vi "Main_Stagefright.vi"() -> ()   [LabVIEW 2012]
uses:
  <vilib>/vision/Image Controls.llb/IMAQ Image.ctl
  <vilib>/vision/NI_Vision_Development_Module.lvlib
panel:
  out "FileVersion":string
  out "Position.y":sgl format="%#.0f"
  out "Position.x":sgl format="%#.0f"
  out "Score":sgl format="%#.0f"
  out "Fiducial Template":T1(plugin-control)
  out "Score all":sgl[](array[numeric])=[207.96088, 1000.0, 164.13931, 159.61043, 129.57571, 190.89413, 153.79263, 159.79875, 217.61157, 150.5897, 141.03848, 539.2585, 523.24445, 511.9799, 522.9404, 526.40063, 548.3722, 524.07715, 509.34766, 529.9397, 530.2488, 546.94275, 528.6569, 540.79004, 501.09125, 521.29175]
  in  "Fiducial Template":string(combo)="Template_20x_sobel.png"
  in  "Save results to CSV":bool
  out "Filename":variant=variant(refnum<image> "StageFrightChip_20x2.bmp")
  out "Source Images":T1[](array[plugin-control])=["20x.bmp", "20x_sobel.bmp", "StageFrightChip_20x.bmp", "StageFrightChip_20x1.bmp", "StageFrightChip_20x2.bmp", "StageFrightChip_20x3.bmp", "StageFrightChip_20x4.bmp", "StageFrightChip_20x5.bmp", "StageFrightChip_20x6.bmp", "StageFrightChip_20x7.bmp", "StageFrightChip_20x8.bmp", "StageFrightChip_20x_sobel.bmp", "StageFrightChip_20x_sobel1.bmp", "StageFrightChip_20x_sobel2.bmp", "StageFrightChip_20x_sobel3.bmp", "StageFrightChip_20x_sobel4.bmp", "StageFrightChip_20x_sobel5.bmp", "StageFrightChip_20x_sobel6.bmp", "StageFrightChip_20x_sobel7.bmp", "StageFrightChip_20x_sobel8.bmp", "StageFrightChip_20x_sobelBright1.bmp", "StageFrightChip_20x_sobelBright2.bmp", "StageFrightChip_20x_sobelBright3.bmp", "StageFrightChip_20x_sobelBright4.bmp", "StageFrightChip_20x_sobelBright5.bmp", "StageFrightChip_20x_sobelBright6.bmp"]
  in  "Size":sgl=10.0
  out "PosY":sgl[](array[numeric])=[1066.1215, 935.5, 484.42477, 541.02295, 617.27484, 638.56024, 1321.046, 729.54535, 897.5891, 1030.7277, 1241.2319, 849.8333, 683.0109, 688.1466, 792.6854, 966.86365, 1146.5382, 1156.1758, 744.771, 868.2035, 868.9183, 866.75134, 866.2604, 1187.9204, 417.75464, 416.24948]
  out "PosX":sgl[](array[numeric])=[1098.6714, 1030.0, 1410.8555, 1155.8539, 1625.7227, 334.02856, 229.2192, 1038.1204, 937.4752, 1740.9315, 435.25806, 1455.6796, 1458.8976, 810.25146, 1064.1396, 1065.0979, 1443.9667, 421.36115, 418.361, 1327.8506, 1331.1934, 1539.8466, 316.55002, 318.59637, 315.33258, 1460.1486]
  in  "Find Patterns":bool
  in  "Folder for Analysis (BMP)":path=path "C:/Users/kevinsh/Desktop/Fiducial Training"
  in  "Overlay Color":u32(colorbox)=16711680
  out "All Results":T1(plugin-control)
  in  "Rotation Angle \nSearch Ranges":cluster{"Start":sgl, "End":sgl}[](array[cluster])=[{"Start"=-10.0, "End"=10.0}]
  in  "Minimum Match Score":sgl=100.0
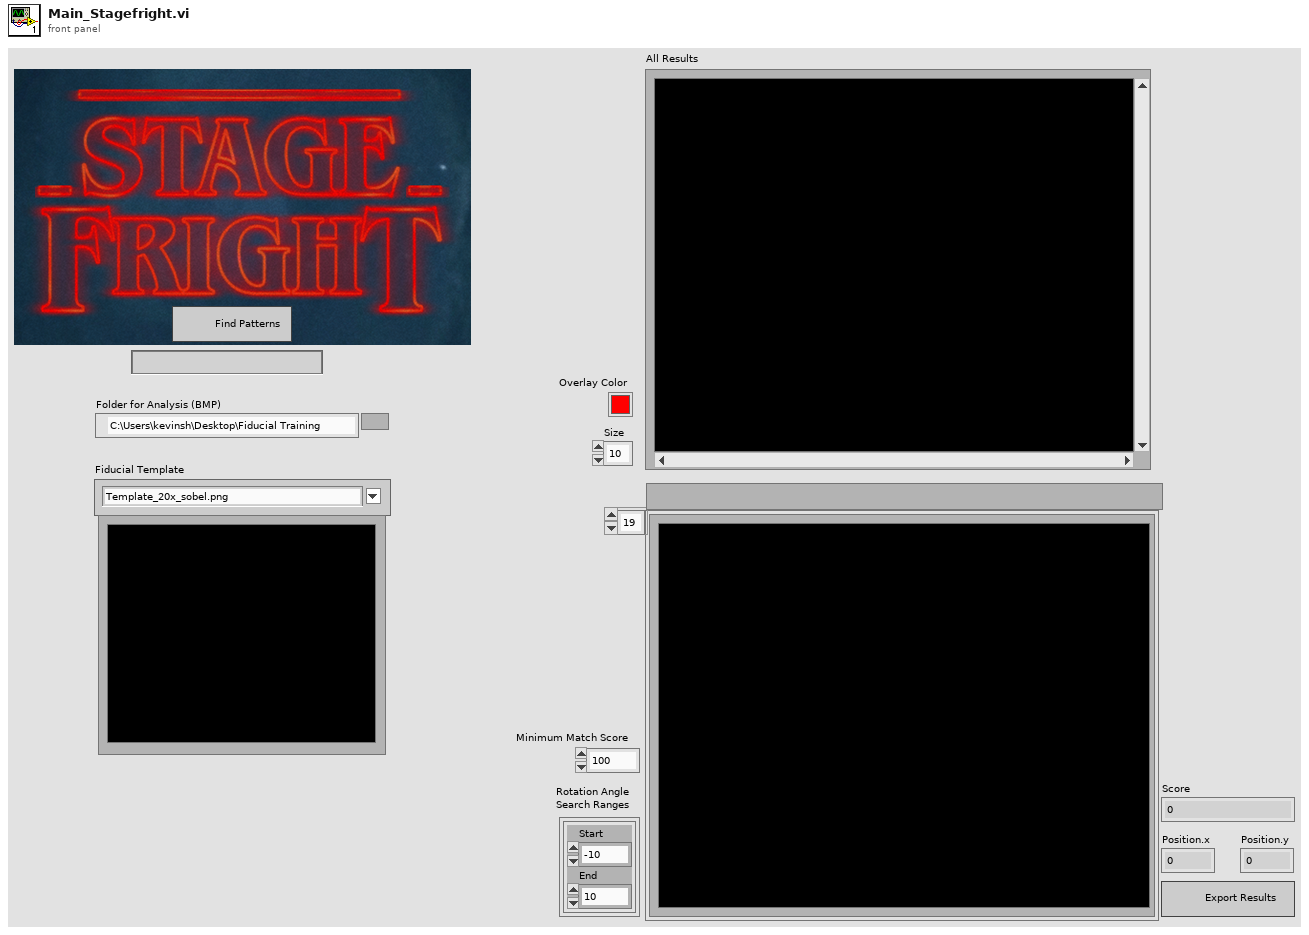
[diagram p1: front panel]
types:
  T1 = typedef "IMAQ Image.ctl" = refnum<image>
  T2 = enum32{"invalid app kind", "Development System", "Run Time System", "Student Edition", "Embedded LabVIEW", "Evaluation", "Custom"}
  T3 = enum32{"Invalid", "Standard", "Closed", "Hidden", "Minimized", "Maximized"}
  T4 = cluster{"Match Mode":u16, "Number of Matches Requested":i32, "Minimum Match Score":sgl, "SubPixel Accuracy":bool, "Rotation Angle Ranges":cluster{"Start":sgl, "End":sgl}[], "Show Search Area":bool, "Show Result":bool}
  T5 = cluster{"Core":cluster{"Current VI Reference":refnum<vi>, "Close Panel on Exit?":bool}, "FiducialImages":T1[], "ImageResults":T1, "PatternTemplate":T1, "PosX":sgl[], "PosY":sgl[], "Score":sgl[], "Folder for Analysis":path, "filenames for processing":string[], "Fiducial Template Path":path, "Data Export Filepath":path}
  T6 = typedef "Image Type" = u32
  T7 = cluster{"Current VI Reference":refnum<vi>, "Close Panel on Exit?":bool}
  T8 = cluster{"Position":cluster{"x":sgl, "y":sgl}, "Angle":sgl, "Scale":sgl, "Score":sgl, "Bounding Box":cluster{"x":sgl, "y":sgl}[]}[]
  T9 = cluster{"Position":cluster{"x":sgl, "y":sgl}, "Angle":sgl, "Scale":sgl, "Score":sgl, "Bounding Box":cluster{"x":sgl, "y":sgl}[]}
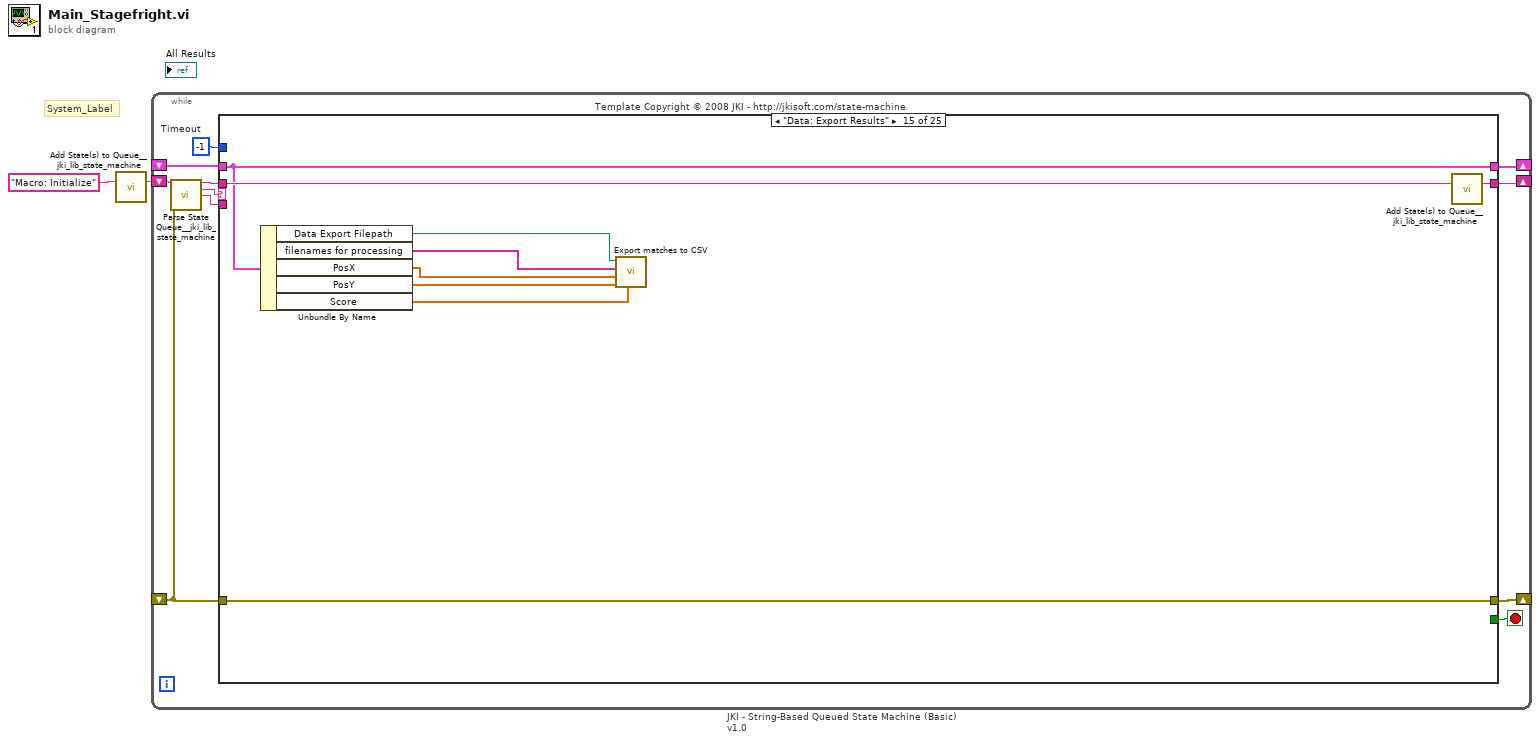
[diagram p0: block diagram]
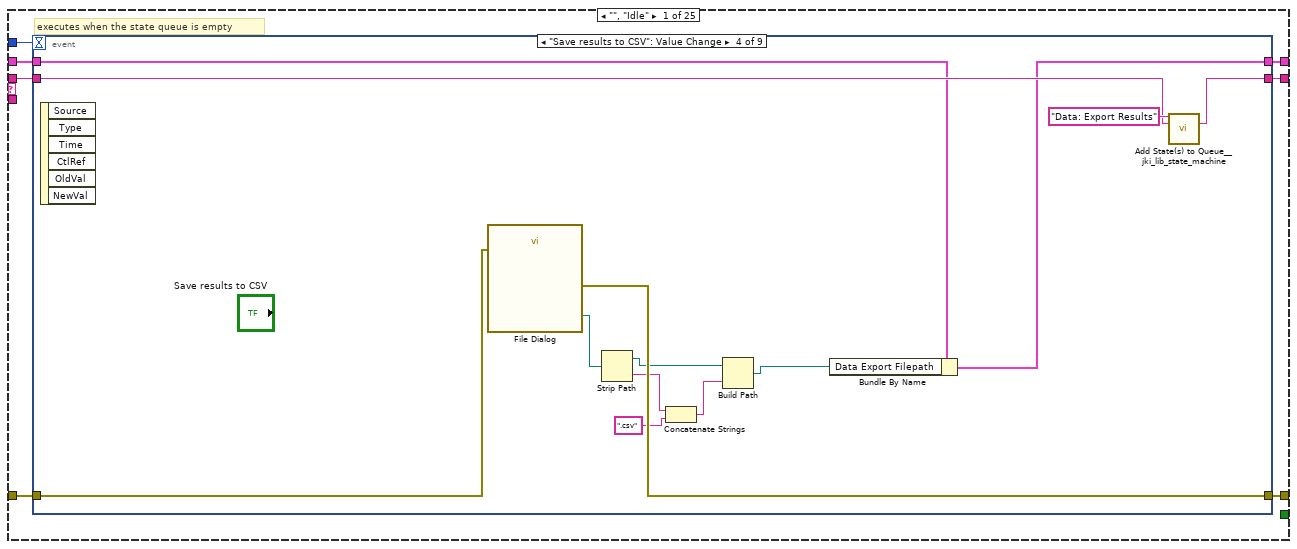
[diagram p2: hidden frame]
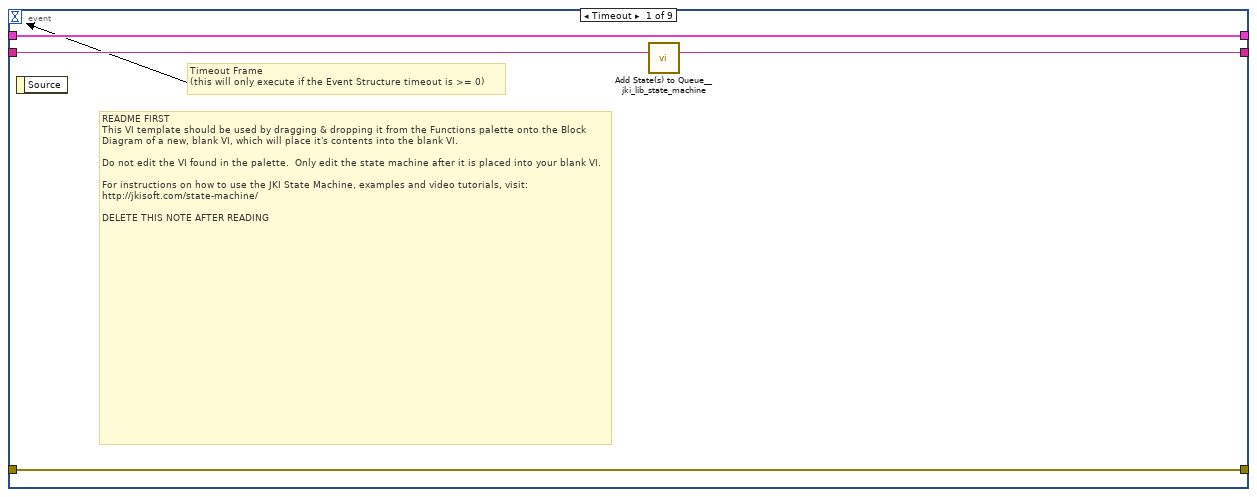
[diagram p3: hidden frame]
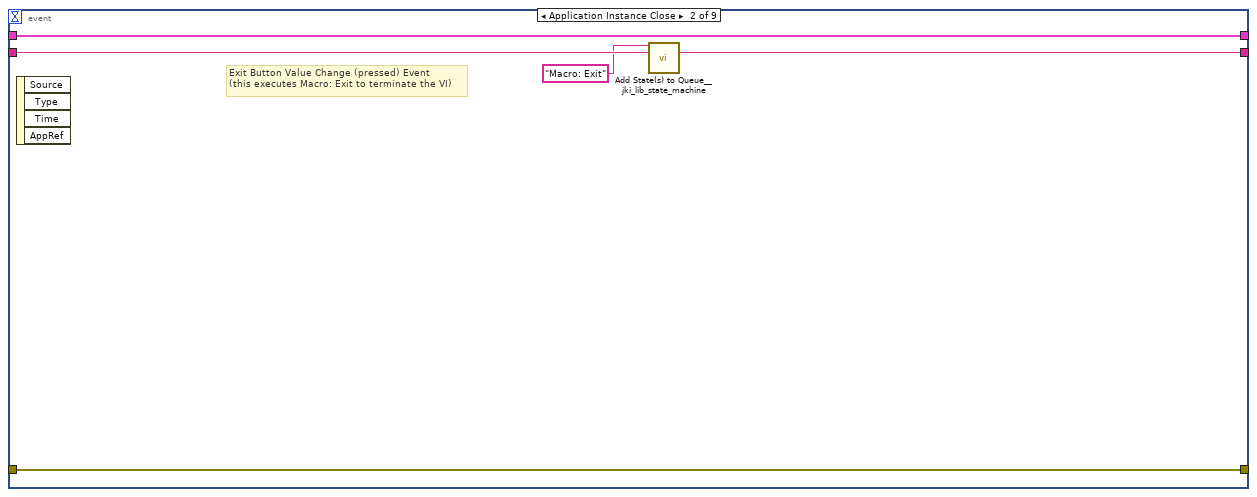
[diagram p4: hidden frame]
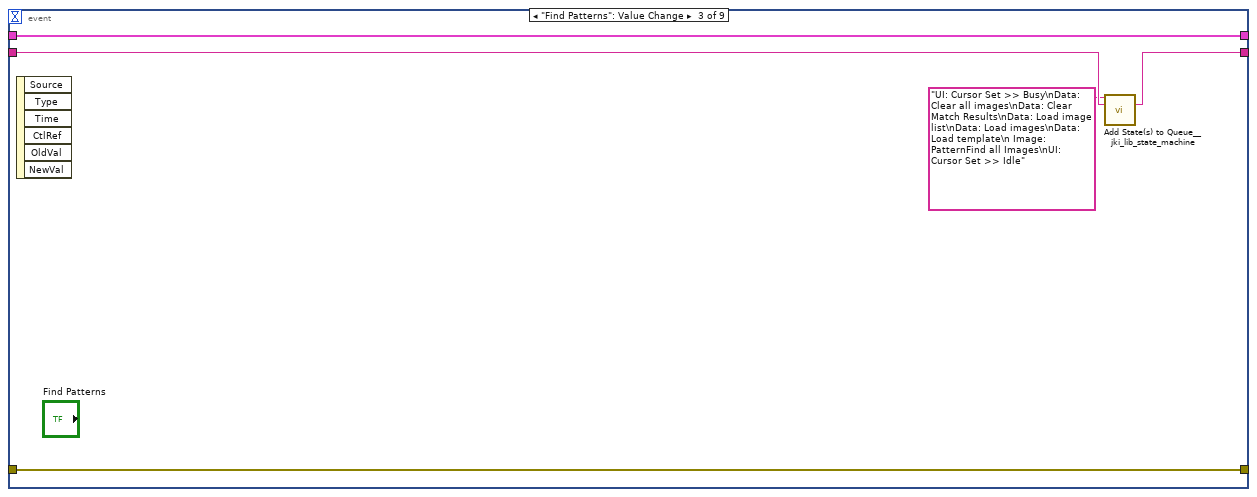
[diagram p5: hidden frame]
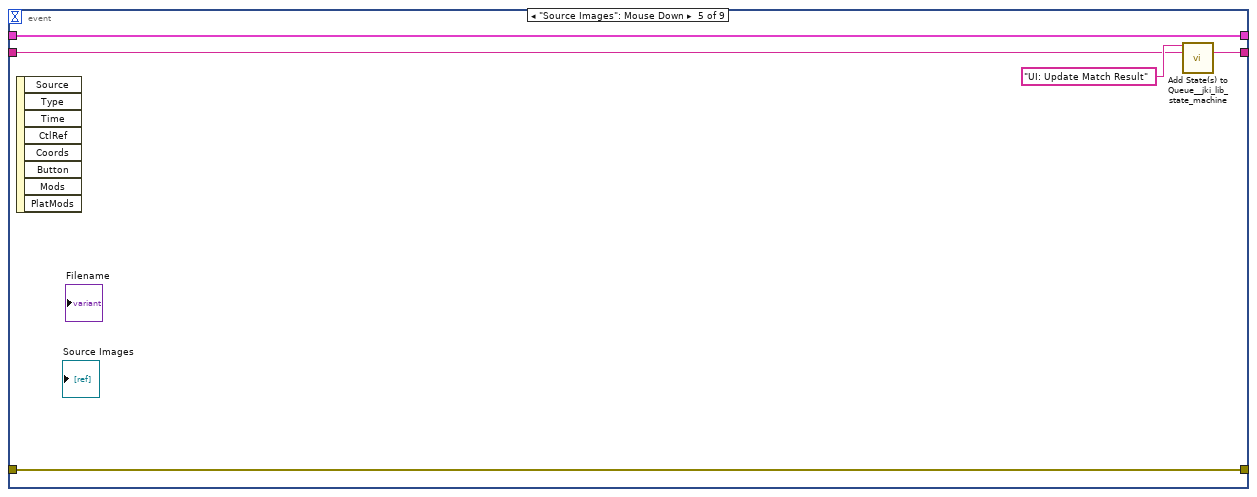
[diagram p6: hidden frame]
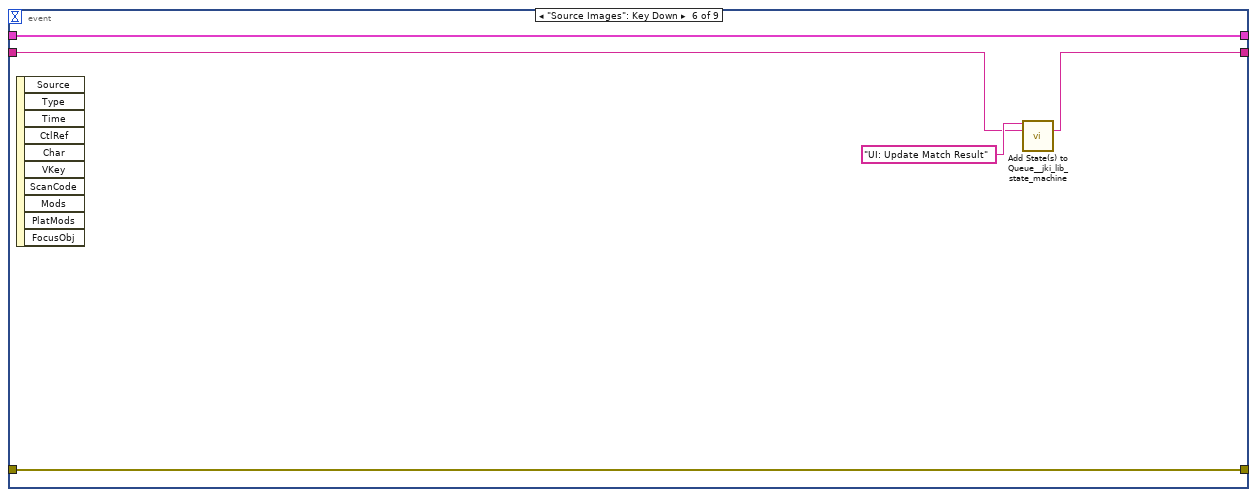
[diagram p7: hidden frame]
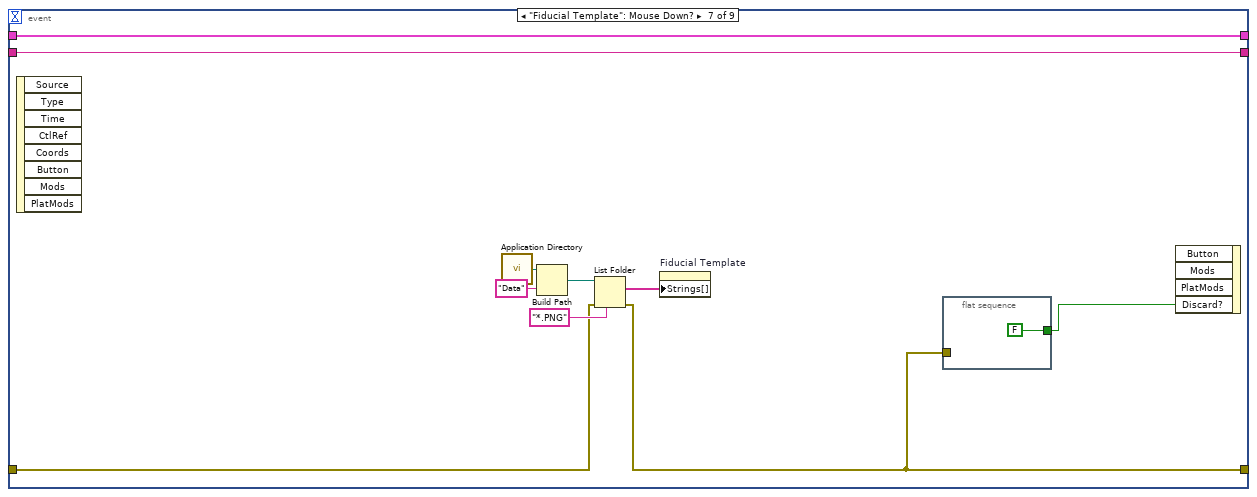
[diagram p8: hidden frame]
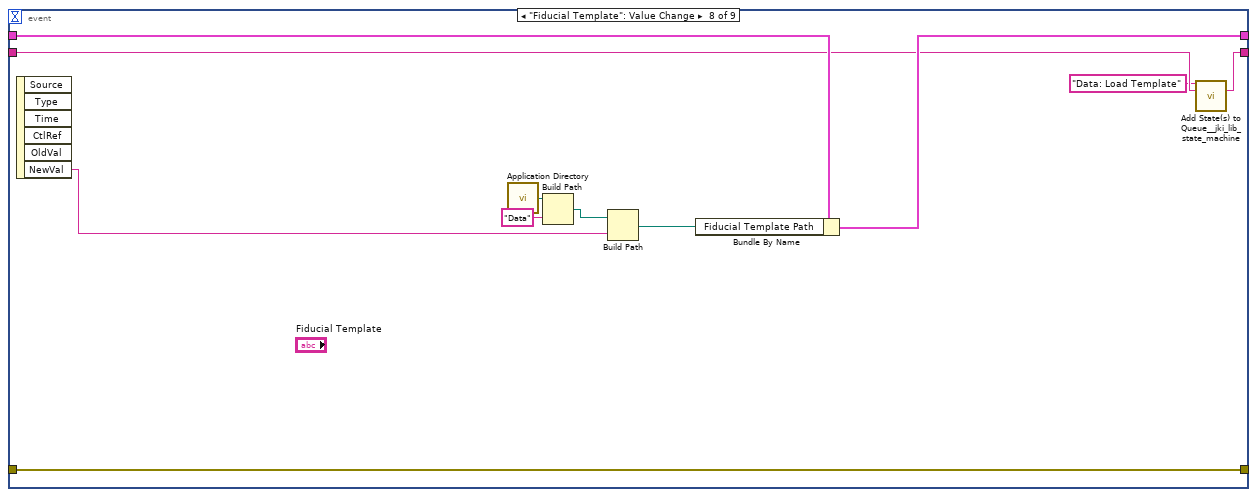
[diagram p9: hidden frame]
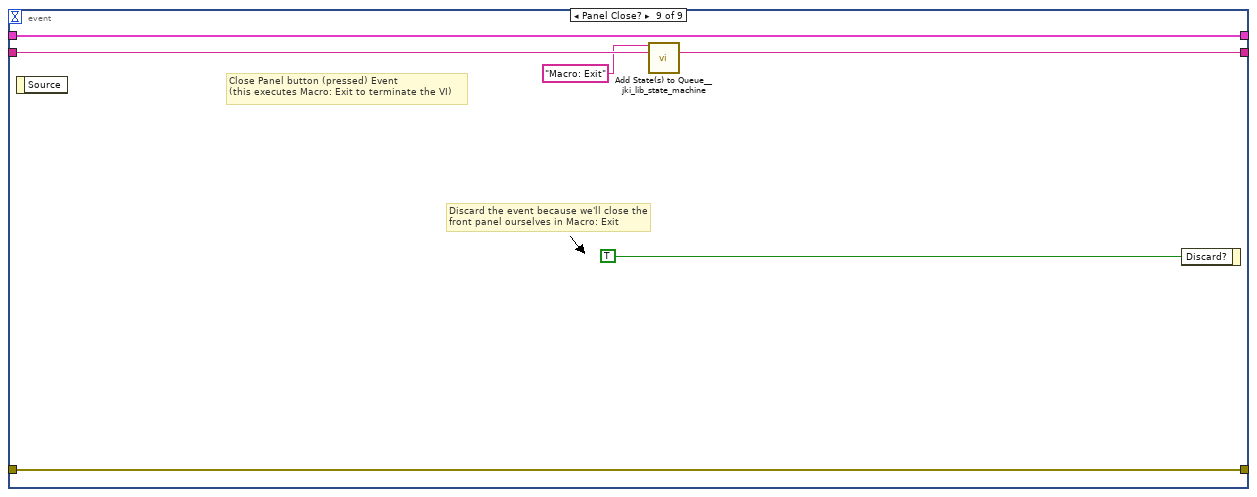
[diagram p10: hidden frame]
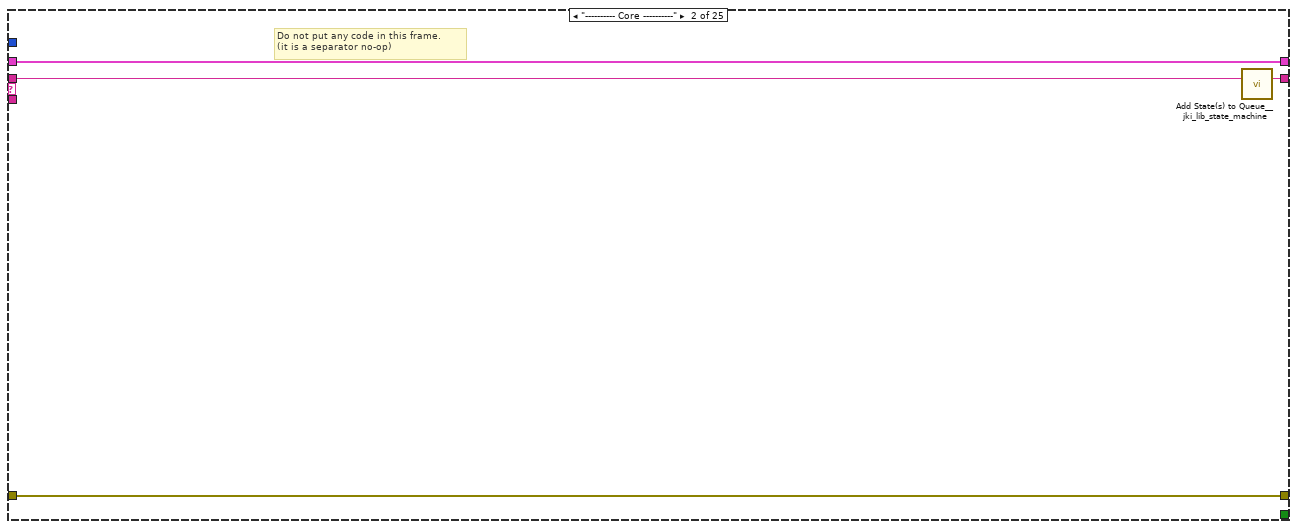
[diagram p11: hidden frame]
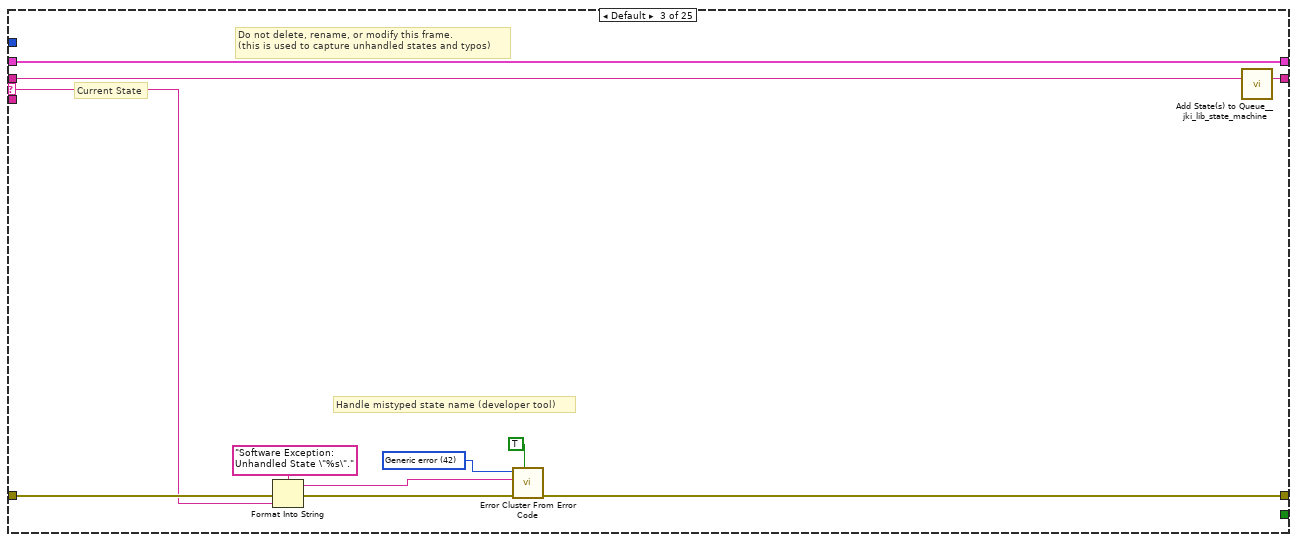
[diagram p12: hidden frame]
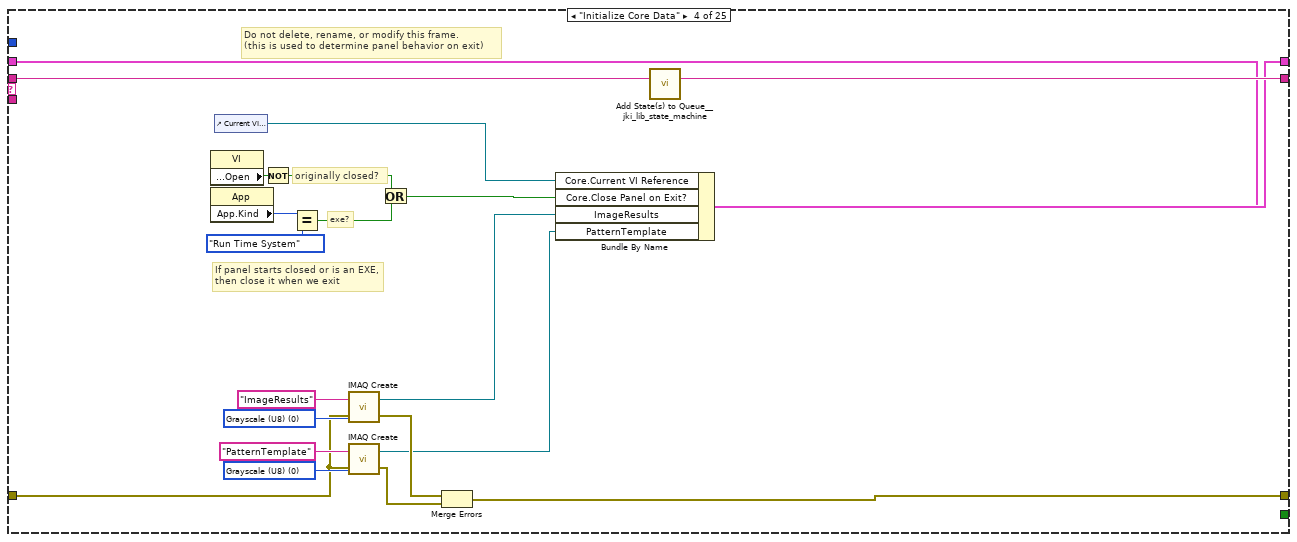
[diagram p13: hidden frame]
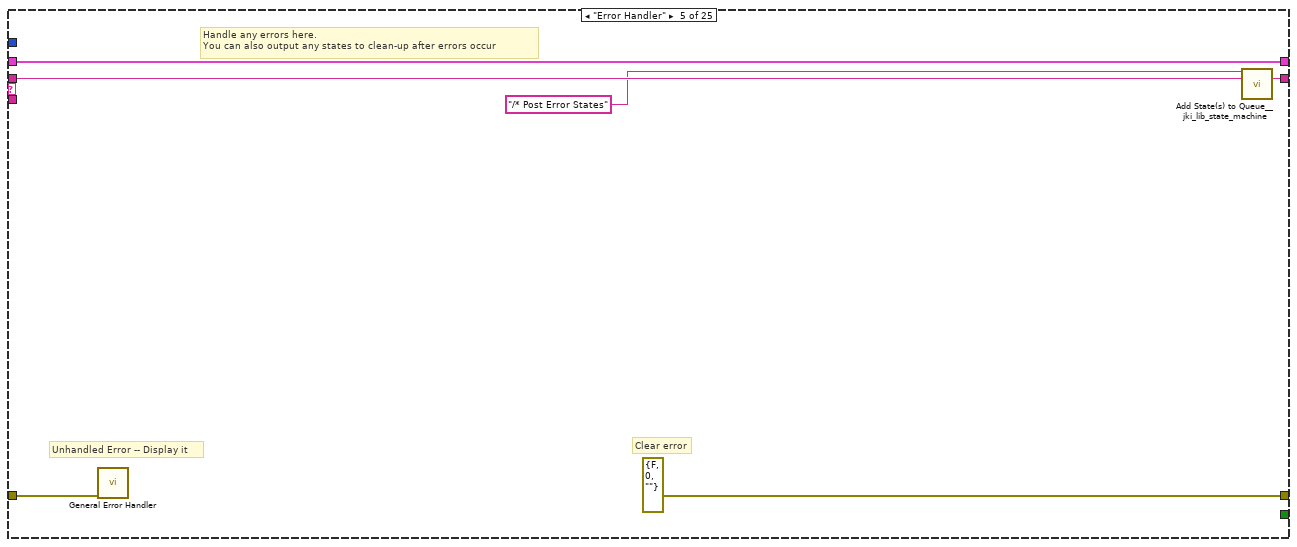
[diagram p14: hidden frame]
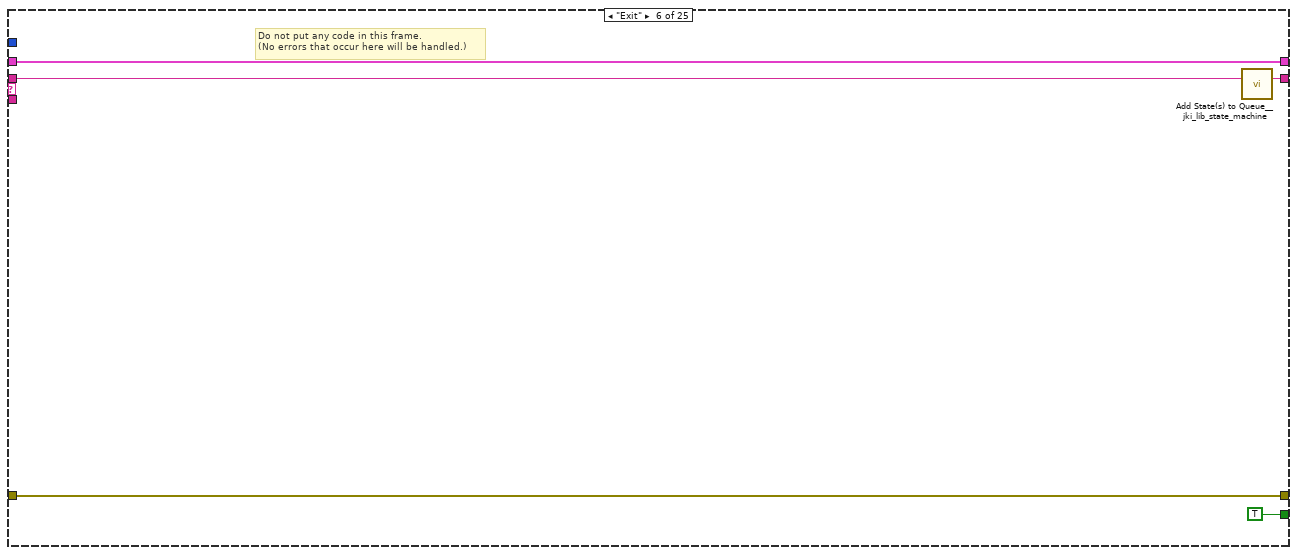
[diagram p15: hidden frame]
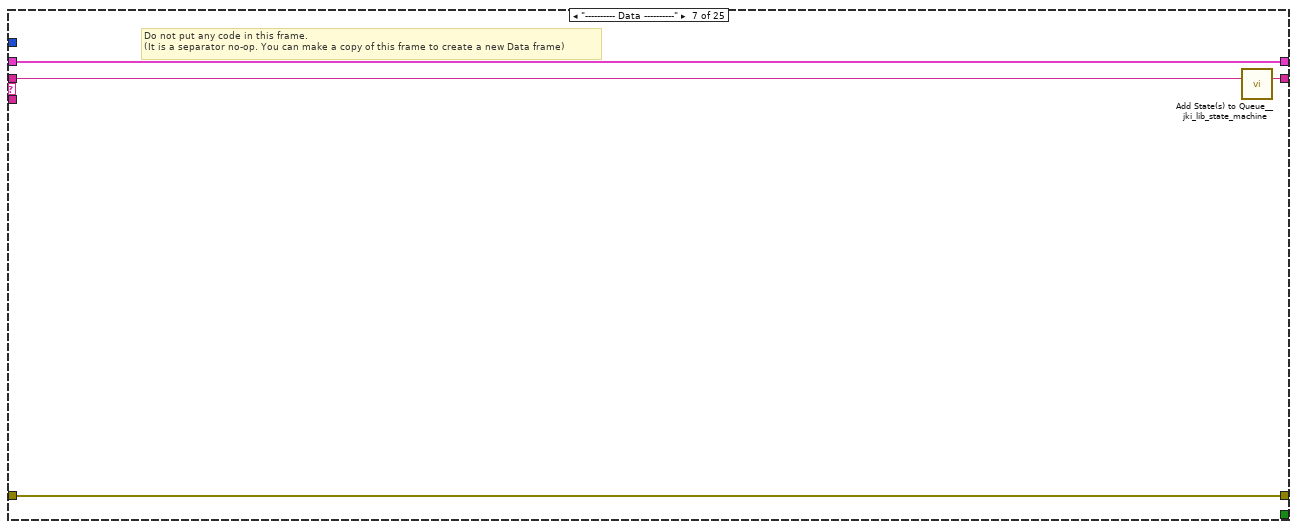
[diagram p16: hidden frame]
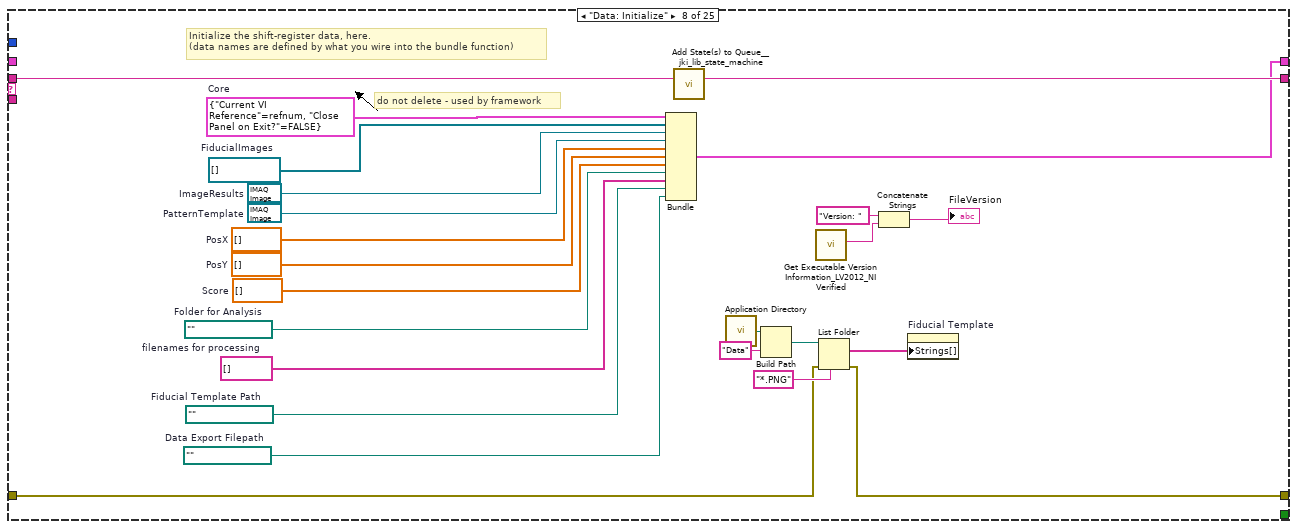
[diagram p17: hidden frame]
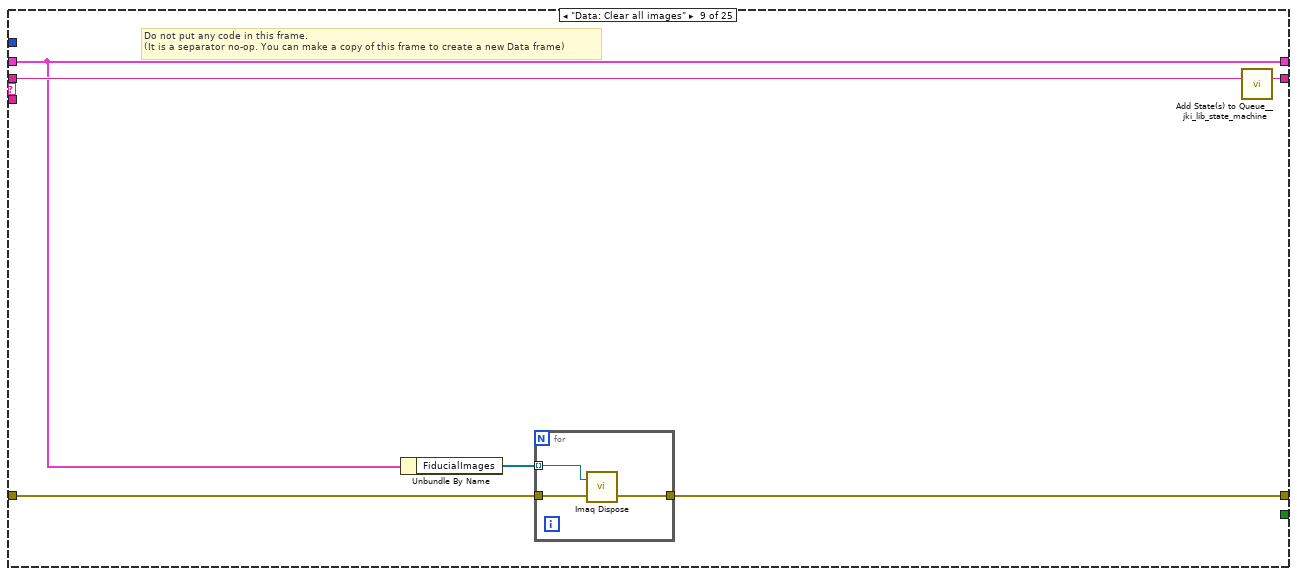
[diagram p18: hidden frame]
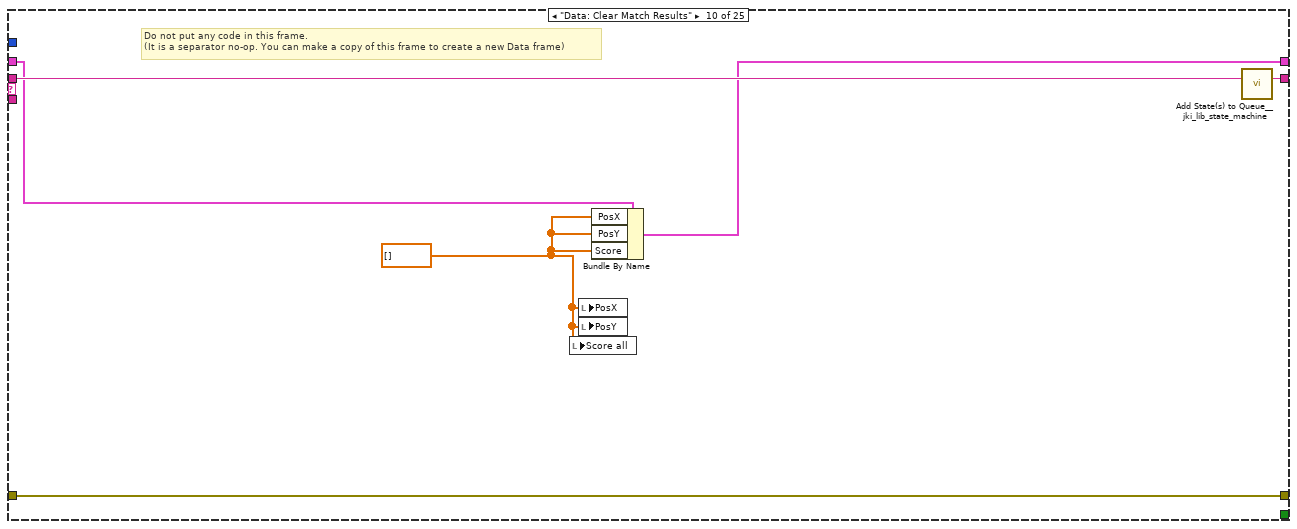
[diagram p19: hidden frame]
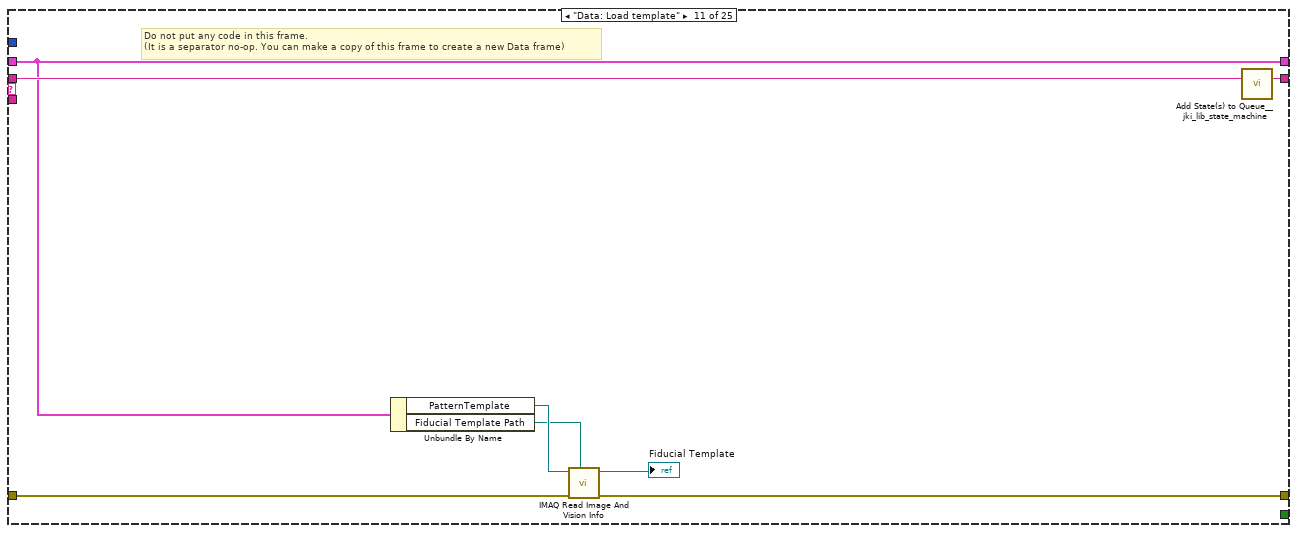
[diagram p20: hidden frame]
diagram:
  # "System_Label"
  n1 = call <vilib>:"Add State(s) to Queue__jki_lib_state_machine.vi"("State(s) in (\"\")"="Macro: Initialize") -> ("States Out"=w2:string)  [unwired: 14 in]
  n2 = while "JKI - String-Based Queued State Machine (Basic) v1.0" {
    shift-right: [w6] -> _
    shift-left: _ -> [w5]
    shift-right: [w9] -> _
    shift-left: _ -> [w3]
    shift-right: [w8] -> _
    shift-left: w2 -> [w10]
    stop <- w7 stop-if-true
    w4 = -1  # Timeout
    # "Template Copyright © 2008 JKI - http://jkisoft.com/state-machine"
    n3 = call <vilib>:"Parse State Queue__jki_lib_state_machine.vi"("State Queue"=w10, "Error In (no error)"=w3) -> ("Remaining States"=w12:string, "Current State"=w13:string, "Arguments"=w11:string)  [unwired: 11 in]
    n4 = case shown="\"Data: Export Results\"" w13 {
      selector: w13 -> [_ _ w90 _ _ _ _ _ _ _ _ _ _ _ _ _ _ _ _ _ _ _ _ _ _]
      tunnel: w12 -> [w20 w89 w94 w121 w127 w132 w136 w160 w166 w175 w183 w192 w204 w222 w231 w235 w248 w252 w258 w269 w295 w300 w310 w314 w335]
      tunnel: w11 -> [_ _ _ _ _ _ _ _ _ _ _ _ _ _ _ _ _ _ w253 w263 _ _ _ _ _]
      tunnel: w5 -> [w18 w86 w92 w113 w124 w130 w133 _ w162 w172 w180 w185 w199 w218 w228 w232 w243 w250 w256 w265 w292 w297 w307 w311 w331]
      tunnel: [w17 w87 w96 w102 errorcluster {"status"=FALSE, "code"=0, "source"=""} ("error out") w129 w134 w143 w163 w173 w178 w186 w196 w219 w229 w233 w246 w249 w254 w266 w293 w298 w308 w312 w325] -> w9
      tunnel: w3 -> [w16 w87 w95 w105 w123 w129 w134 w144 w164 w173 w179 w187 w202 w216 w229 w233 w246 w249 w255 w267 w293 w298 w308 w312 w333]
      tunnel: [w19 w88 w93 w120 w126 w131 w135 w159 w165 w174 w182 w191 w203 w221 w230 w234 w247 w251 w257 w268 w294 w299 w309 w313 w334] -> w8
      tunnel: [_ _ _ _ _ TRUE _ _ _ _ _ _ _ _ _ _ _ _ _ _ _ _ _ _ _] -> w7
      tunnel: [w15 w86 w92 w119 w124 w130 w133 w158 w162 w171 w180 w184 w198 w218 w228 w232 w243 w250 w256 w265 w292 w297 w307 w311 w329] -> w6
      tunnel: w4 -> [w14 _ _ _ _ _ _ _ _ _ _ _ _ _ _ _ _ _ _ _ _ _ _ _ _]
      frame "", "Idle" {
        # "executes when the state queue is empty"
        n5 = event shown="[3] \"Save results to CSV\": Value Change" {
          selector: _ -> [_ _ _ _ _ _ _ _ _]
          dyn-events: _ -> [_ _ _ _ _ _ _ _ _]
          timeout: w14 -> [_ _ _ _ _ _ _ _ _]
          tunnel: w20 -> [w24 w29 w32 w46 w49 w54 w67 w70 w85]
          tunnel: [w23 w28 w31 w45 w48 w53 w67 w71 w84] -> w19
          tunnel: w18 -> [w21 w26 w33 w42 w51 w56 w66 w77 w82]
          tunnel: [w22 w27 w34 w43 w52 w57 w58 w79 w83] -> w17
          tunnel: w16 -> [w22 w27 w34 w44 w52 w57 w60 w79 w83]
          tunnel: [w21 w26 w33 w41 w51 w56 w66 w76 w82] -> w15
          event Timeout {
            # "README FIRST\nThis VI template should be used by dragging & dropping it from the Functions palette onto the Block Diagram of a new, blank VI, which will place it's contents into the blank VI.\n\nDo not edit the VI found in the palette.  Only edit the state machine after it is placed into your blank VI.\n\nFor instructions on how to use the JKI State Machine, examples and video tutorials, visit:\nhttp://jkisoft.com/state-machine/\n\nDELETE THIS NOTE AFTER READING"
            # "Timeout Frame\n(this will only execute if the Event Structure timeout is >= 0)"
            n6 = event-data() -> ()  [unwired: 1 in, 1 out]
            n7 = call <vilib>:"Add State(s) to Queue__jki_lib_state_machine.vi"("State(s) in (\"\")"=w24) -> ("States Out"=w23:string)  [unwired: 14 in]
          }
          event Application Instance Close {
            # "Exit Button Value Change (pressed) Event\n(this executes Macro: Exit to terminate the VI)"
            n8 = event-data() -> ()  [unwired: 1 in, 4 out]
            n9 = call <vilib>:"Add State(s) to Queue__jki_lib_state_machine.vi"("State(s) in Front (\"\")"="Macro: Exit", "State(s) in (\"\")"=w29) -> ("States Out"=w28:string)  [unwired: 13 in]
          }
          event "Find Patterns": Value Change {
            n10 = event-data() -> ()  [unwired: 1 in, 6 out]
            n11 = call <vilib>:"Add State(s) to Queue__jki_lib_state_machine.vi"("State(s) in Front (\"\")"="UI: Cursor Set >> Busy\nData: Clear all images\nData: Clear Match Results\nData: Load image list\nData: Load images\nData: Load template\n Image: PatternFind all Images\nUI: Cursor Set >> Idle" ("State(s) in Front (\"\")"), "State(s) in (\"\")"=w32) -> ("States Out"=w31:string)  [unwired: 13 in]
          }
          event "Save results to CSV": Value Change {
            n12 = event-data() -> ()  [unwired: 1 in, 6 out]
            n13 = call "File Dialog"("error in"=w44) -> ("selected path"=w40:path, "error out"=w43:errorcluster)  [unwired: 11 in, 2 out]
            n14 = Strip Path(path=w40) -> (stripped path=w39:path, name=w38:string)
            n15 = Concatenate Strings(w38, ".csv" ("name or relative path")) -> (w36:string)
            n16 = Build Path(base path=w39, name or relative path=w36) -> (appended path=w35:path)
            n17 = Bundle By Name(cluster=w42, "Data Export Filepath"=w35) -> (w41:T5)
            n18 = call <vilib>:"Add State(s) to Queue__jki_lib_state_machine.vi"("State(s) in Front (\"\")"="Data: Export Results" ("State(s) in Front (\"\")"), "State(s) in (\"\")"=w46) -> ("States Out"=w45:string)  [unwired: 13 in]
          }
          event "Source Images": Mouse Down {
            n19 = event-data() -> ()  [unwired: 1 in, 8 out]
            n20 = call <vilib>:"Add State(s) to Queue__jki_lib_state_machine.vi"("State(s) in Front (\"\")"="UI: Update Match Result", "State(s) in (\"\")"=w49) -> ("States Out"=w48:string)  [unwired: 13 in]
          }
          event "Source Images": Key Down {
            n21 = event-data() -> ()  [unwired: 1 in, 10 out]
            n22 = call <vilib>:"Add State(s) to Queue__jki_lib_state_machine.vi"("State(s) in Front (\"\")"="UI: Update Match Result", "State(s) in (\"\")"=w54) -> ("States Out"=w53:string)  [unwired: 13 in]
          }
          event "Fiducial Template": Mouse Down? {
            n23 = event-data() -> ()  [unwired: 1 in, 8 out]
            n24 = call <vilib>:"Application Directory.vi"() -> ("Application Directory"=w64:path)
            n25 = Build Path(base path=w64, name or relative path="Data") -> (appended path=w65:path)
            n26 = List Folder(path=w65, pattern="*.PNG", error in=w60) -> (filenames=w62:string[], error out=w58:errorcluster)  [unwired: 1 in, 2 out]
            n27 = property on="Fiducial Template" class="CmbBox"("Strings[]"=w62) -> ()  [unwired: 2 in, 2 out]
            n28 = flat-sequence {
              tunnel: [FALSE ("Discard?")] -> w59
              tunnel: w58 -> [_]
              frame #0 {
              }
            }
            n29 = event-data("Discard?"=w59) -> ()  [unwired: 4 in, 1 out]
          }
          event "Fiducial Template": Value Change {
            n30 = event-data() -> ("NewVal"=w78:string)  [unwired: 1 in, 5 out]
            n31 = call <vilib>:"Application Directory.vi"() -> ("Application Directory"=w74:path)
            n32 = Build Path(base path=w74, name or relative path="Data") -> (appended path=w72:path)
            n33 = Build Path(base path=w72, name or relative path=w78) -> (appended path=w75:path)
            n34 = Bundle By Name(cluster=w77, "Fiducial Template Path"=w75) -> (w76:T5)
            n35 = call <vilib>:"Add State(s) to Queue__jki_lib_state_machine.vi"("State(s) in Front (\"\")"="Data: Load Template" ("State(s) in Front (\"\")"), "State(s) in (\"\")"=w70) -> ("States Out"=w71:string)  [unwired: 13 in]
          }
          event Panel Close? {
            # "Discard the event because we'll close the front panel ourselves in Macro: Exit"
            # "Close Panel button (pressed) Event\n(this executes Macro: Exit to terminate the VI)"
            n36 = event-data() -> ()  [unwired: 1 in, 1 out]
            n37 = call <vilib>:"Add State(s) to Queue__jki_lib_state_machine.vi"("State(s) in Front (\"\")"="Macro: Exit", "State(s) in (\"\")"=w85) -> ("States Out"=w84:string)  [unwired: 13 in]
            n38 = event-data("Discard?"=TRUE) -> ()  [unwired: 1 in, 1 out]
          }
        }
      }
      frame "---------- Core ----------" {
        # "Do not put any code in this frame.\n(it is a separator no-op)"
        n39 = call <vilib>:"Add State(s) to Queue__jki_lib_state_machine.vi"("State(s) in (\"\")"=w89) -> ("States Out"=w88:string)  [unwired: 14 in]
      }
      frame Default {
        w99 = 42 items=["No error", "Argument error", "Memory is full", "Out of zone", "End of file", "File already open", "Generic file I/O error", "File not found", "File permission error", "Disk is full", "Duplicate path", "Too many files open", "System feature not enabled", "Resource file not found", "Cannot add resource", "Resource not found", "Image not found", "Image memory error", "Pen does not exist", "Config type invalid", "Config token not found", "Config parse error", "Config memory error", "Bad external code format", "Bad external code offset", "External code not present", "Null window", "Destroy window error", "Null menu", "Print aborted", "Bad print record", "Print driver error", "Windows error during printing", "Memory error during printing", "Print dialog error", "Generic print error", "Invalid device refnum", "Device not found", "Device parameter error", "Device unit error", "Cannot open device", "Device call aborted", "Generic error", "Cancelled by user", "Object ID too low", "Object ID too high", "Object not in heap", "Unknown heap", "Unknown object (invalid DefProc)", "Unknown object (DefProc not in table)", "Message out of range", "Invalid (null) method", "Unknown message", "Manager call not supported", "Bad address", "Network operation in progress", "Network operation timed out", "Connection is busy", "Network attribute not supported", "Network error", "Address in use", "System out of memory", "Connection aborted", "Connection refused", "Not connected", "Already connected", "Connection closed", "Initialization error (interapplication manager)", "Bad occurrence", "Wait on unbound occurrence handler", "Occurrence queue overflow", "Datalog type conflict", "Unused", "Unrecognized type (interapplication manager)", "Memory corrupt", "Failed to make temporary DLL", "Old CIN version", "Drag socket not found", "Failed to load drop-object", "Failed to register OLE object", "Failed to release OLE object", "Format specifier type mismatch", "Unknown format specifier", "Too few format specifiers", "Too many format specifiers", "Scan failed", "Newer CIN version", "Error converting to variant", "Runtime menu error", "Password tampered", "Variant attribute not found", "Incompatible variant data type", "Event data is not available", "Event Store is not present", "Occurrence is not found", "Event Queue is not created", "Event info is not available", "Refnum passed is NULL", "Error retrieving Class GUID", "Error retrieving CoClass GUID", "Error retrieving TypeLib GUID.", "Bad built application magic bytes.", "Specific driver is different from the specific driver associated with the Logical Name.", "There is no session opened to the class driver.", "Max Error", "MAX - Error with config objects", "MAX - Error loading configuration", "MAX - Group not supported"]
        # "Current State"
        # "Do not delete, rename, or modify this frame.\n(this is used to capture unhandled states and typos)"
        # "Handle mistyped state name (developer tool)"
        n40 = Format Into String(format string="Software Exception: Unhandled State \"%s\"." ("message"), error in=w95, w90) -> (resulting string=w98:string, error out=w97:errorcluster)  [unwired: 1 in]
        n41 = call <vilib>:"Error Cluster From Error Code.vi"("show call chain? (False)"=TRUE, "error in (no error)"=w97, "error message (\"\")"=w98, "error code (0)"=w99) -> ("error out"=w96:errorcluster)  [unwired: 5 in]
        n42 = call <vilib>:"Add State(s) to Queue__jki_lib_state_machine.vi"("State(s) in (\"\")"=w94) -> ("States Out"=w93:string)  [unwired: 14 in]
      }
      frame "Initialize Core Data" {
        w107 = T6 0 items=["Grayscale (U8)", "Grayscale (I16)", "Grayscale (SGL)", "Complex (CSG)", "RGB (U32)", "HSL (U32)", "RGB (U64)", "Grayscale (U16)"] ("Image Type")
        w109 = T6 0 items=["Grayscale (U8)", "Grayscale (I16)", "Grayscale (SGL)", "Complex (CSG)", "RGB (U32)", "HSL (U32)", "RGB (U64)", "Grayscale (U16)"] ("Image Type")
        # "Do not delete, rename, or modify this frame.\n(this is used to determine panel behavior on exit)"
        # "originally closed?"
        # "exe?"
        # "If panel starts closed or is an EXE, then close it when we exit"
        n43 = property class="VI"() -> ("Front Panel.Open"=w118:bool)  [unwired: 2 in, 2 out]
        n44 = property class="App"() -> ("App.Kind"=w117:T2)  [unwired: 2 in, 2 out]
        n45 = control-ref of="Current VI Reference"() -> (w111:refnum<vi>)
        n46 = Not(x=w118) -> (.not. x?=w115:bool)
        n47 = Equal?(x=w117, y=T2."Run Time System" ("Application:Kind")) -> (x = y?=w114:bool)
        n48 = call "IMAQ Create"("Image Name"="ImageResults", "Image Type"=w109, "error in (no error)"=w105) -> ("New Image"=w108:T1, "error out"=w104:errorcluster)  [unwired: 1 in, 1 out]
        n49 = call "IMAQ Create"("Image Name"="PatternTemplate", "Image Type"=w107, "error in (no error)"=w105) -> ("New Image"=w101:T1, "error out"=w103:errorcluster)  [unwired: 1 in, 1 out]
        n50 = Or(x=w115, y=w114) -> (x .or. y?=w112:bool)
        n51 = Merge Errors(w104, w103) -> (w102:errorcluster)
        n52 = Bundle By Name(cluster=w113, "Core.Current VI Reference"=w111, "Core.Close Panel on Exit?"=w112, "ImageResults"=w108, "PatternTemplate"=w101) -> (w119:T5)
        n53 = call <vilib>:"Add State(s) to Queue__jki_lib_state_machine.vi"("State(s) in (\"\")"=w121) -> ("States Out"=w120:string)  [unwired: 14 in]
      }
      frame "Error Handler" {
        # "Unhandled Error -- Display it"
        # "Handle any errors here.\nYou can also output any states to clean-up after errors occur"
        # "Clear error"
        n54 = call <vilib>:"General Error Handler.vi"("error in (no error)"=w123) -> ()  [unwired: 10 in, 5 out]
        n55 = call <vilib>:"Add State(s) to Queue__jki_lib_state_machine.vi"("State(s) in Front (\"\")"="/* Post Error States", "State(s) in (\"\")"=w127) -> ("States Out"=w126:string)  [unwired: 13 in]
      }
      frame "Exit" {
        # "Do not put any code in this frame.\n(No errors that occur here will be handled.)"
        n56 = call <vilib>:"Add State(s) to Queue__jki_lib_state_machine.vi"("State(s) in (\"\")"=w132) -> ("States Out"=w131:string)  [unwired: 14 in]
      }
      frame "---------- Data ----------" {
        # "Do not put any code in this frame.\n(It is a separator no-op. You can make a copy of this frame to create a new Data frame)"
        n57 = call <vilib>:"Add State(s) to Queue__jki_lib_state_machine.vi"("State(s) in (\"\")"=w136) -> ("States Out"=w135:string)  [unwired: 14 in]
      }
      frame "Data: Initialize" {
        w140 = path ""  # Data Export Filepath
        w141 = sgl[] []  # Score
        w149 = path ""  # Fiducial Template Path
        w150 = T1[] []  # FiducialImages
        w151 = string[] []  # filenames for processing
        w152 = path ""  # Folder for Analysis
        w153 = sgl[] []  # PosY
        w154 = sgl[] []  # PosX
        w155 = T1 refnum  # PatternTemplate
        w156 = T1 refnum  # ImageResults
        w157 = T7 {"Current VI Reference"=refnum, "Close Panel on Exit?"=FALSE}  # Core
        # "do not delete - used by framework"
        # "Initialize the shift-register data, here.\n(data names are defined by what you wire into the bundle function)"
        n58 = Bundle("Core"=w157, "FiducialImages"=w150, "ImageResults"=w156, "PatternTemplate"=w155, "PosX"=w154, "PosY"=w153, "Score"=w141, "Folder for Analysis"=w152, "filenames for processing"=w151, "Fiducial Template Path"=w149, "Data Export Filepath"=w140) -> (w158:T5)  [unwired: 1 in]
        n59 = call <vilib>:"Add State(s) to Queue__jki_lib_state_machine.vi"("State(s) in (\"\")"=w160) -> ("States Out"=w159:string)  [unwired: 14 in]
        n60 = call <vilib>:"Application Directory.vi"() -> ("Application Directory"=w147:path)
        n61 = Build Path(base path=w147, name or relative path="Data") -> (appended path=w148:path)
        n62 = call "Get Executable Version Information_LV2012_NI Verified.vi"() -> ("FileVersion"=w137:string)  [unwired: 10 in, 1 out]
        n63 = List Folder(path=w148, pattern="*.PNG", error in=w144) -> (filenames=w142:string[], error out=w143:errorcluster)  [unwired: 1 in, 2 out]
        n64 = Concatenate Strings("Version: " ("string"), w137) -> (→"FileVersion":string)
        n65 = property on="Fiducial Template" class="CmbBox"("Strings[]"=w142) -> ()  [unwired: 2 in, 2 out]
      }
      frame "Data: Clear all images" {
        # "Do not put any code in this frame.\n(It is a separator no-op. You can make a copy of this frame to create a new Data frame)"
        n66 = Unbundle By Name(w162) -> ("FiducialImages"=w161:T1[])
        n67 = for {
          tunnel: w164 -> [w169]
          tunnel: [w168] -> w163
          tunnel: w161 -> [w167] mode=indexing
          n68 = call "Imaq Dispose"("Image"=w167, "error in (no error)"=w169) -> ("error out"=w168:errorcluster)  [unwired: 4 in]
        }
        n69 = call <vilib>:"Add State(s) to Queue__jki_lib_state_machine.vi"("State(s) in (\"\")"=w166) -> ("States Out"=w165:string)  [unwired: 14 in]
      }
      frame "Data: Clear Match Results" {
        w170 = sgl[] [] ("PosX")
        # "Do not put any code in this frame.\n(It is a separator no-op. You can make a copy of this frame to create a new Data frame)"
        n70 = local write "Score all"(w170) -> ()
        n71 = local write "PosX"(w170) -> ()
        n72 = local write "PosY"(w170) -> ()
        n73 = Bundle By Name(cluster=w172, "PosX"=w170, "PosY"=w170, "Score"=w170) -> (w171:T5)
        n74 = call <vilib>:"Add State(s) to Queue__jki_lib_state_machine.vi"("State(s) in (\"\")"=w175) -> ("States Out"=w174:string)  [unwired: 14 in]
      }
      frame "Data: Load template" {
        # "Do not put any code in this frame.\n(It is a separator no-op. You can make a copy of this frame to create a new Data frame)"
        n75 = Unbundle By Name(w180) -> ("PatternTemplate"=w181:T1, "Fiducial Template Path"=w177:path)
        n76 = call "IMAQ Read Image And Vision Info"("File Path"=w177, "error in (no error)"=w179, "Image"=w181) -> ("error out"=w178:errorcluster, "Image Out"=→"Fiducial Template":T1)  [unwired: 1 in, 6 out]
        n77 = call <vilib>:"Add State(s) to Queue__jki_lib_state_machine.vi"("State(s) in (\"\")"=w183) -> ("States Out"=w182:string)  [unwired: 14 in]
      }
      frame "Data: Load image list" {
        n78 = List Folder(path="Folder for Analysis (BMP)", pattern="*.BMP", error in=w187) -> (filenames=w189:string[], error out=w186:errorcluster)  [unwired: 1 in, 2 out]
        n79 = in-place {
          in-place-border: w189 -> [w194]
          in-place-border: "Folder for Analysis (BMP)" -> [w193]
          n80 = in-place-cluster #1(w185) -> ()  [unwired: 2 out]
          n81 = in-place-cluster #1("Folder for Analysis"=w193, "filenames for processing"=w194) -> (w184:T5)
        }
        n82 = call <vilib>:"Add State(s) to Queue__jki_lib_state_machine.vi"("State(s) in (\"\")"=w192) -> ("States Out"=w191:string)  [unwired: 14 in]
      }
      frame "Data: Load images" {
        n83 = Unbundle By Name(w199) -> ("Folder for Analysis"=w201:path, "filenames for processing"=w200:string[])
        n84 = for {
          shift-right: [w214] -> w196
          shift-left: w202 -> [w211]
          tunnel: w201 -> [w213]
          tunnel: w200 -> [w208] mode=indexing
          tunnel: [w212] -> w197 mode=indexing
          tunnel: [w205] -> w195 mode=indexing
          w207 = T6 0 items=["Grayscale (U8)", "Grayscale (I16)", "Grayscale (SGL)", "Complex (CSG)", "RGB (U32)", "HSL (U32)", "RGB (U64)", "Grayscale (U16)"] ("Image Type")
          n85 = call "IMAQ Create"("Image Name"=w208, "Image Type"=w207, "error in (no error)"=w211) -> ("New Image"=w209:T1, "error out"=w210:errorcluster)  [unwired: 2 in]
          n86 = Build Path(base path=w213, name or relative path=w208) -> (appended path=w206:path)
          n87 = call "IMAQ ReadFile"("File Path"=w206, "error in (no error)"=w210, "Image"=w209) -> ("error out"=w214:errorcluster, "Image Out"=w212:T1)  [unwired: 4 in, 3 out]
          n88 = call <vilib>:"Get File Extension.vi"("file"=w206) -> ("filename without extension"=w205:string)  [unwired: 7 in, 3 out]
        }
        n89 = Bundle By Name(cluster=w199, "filenames for processing"=w195, "FiducialImages"=w197) -> (w198:T5)
        n90 = call <vilib>:"Add State(s) to Queue__jki_lib_state_machine.vi"("State(s) in (\"\")"=w204) -> ("States Out"=w203:string)  [unwired: 14 in]
      }
      frame "Data: Cleanup" {
        # "Cleanup any data and references, here.\n(this is called automatically, by the Macro: Exit)"
        n91 = Unbundle By Name(w218) -> ("Core.Current VI Reference"=w220:refnum<vi>)
        n92 = call "Imaq Dispose"("All Images? (No)"=TRUE, "error in (no error)"=w216) -> ("error out"=w215:errorcluster)  [unwired: 4 in]
        n93 = Close Reference(reference=w220, error in (no error)=w215) -> (error out=w219:errorcluster)
        n94 = call <vilib>:"Add State(s) to Queue__jki_lib_state_machine.vi"("State(s) in (\"\")"=w222) -> ("States Out"=w221:string)  [unwired: 14 in]
      }
      frame "Data: Export Results" {
        n95 = Unbundle By Name(w228) -> ("Data Export Filepath"=w223:path, "filenames for processing"=w224:string[], "PosX"=w227:sgl[], "PosY"=w226:sgl[], "Score"=w225:sgl[])
        n96 = call "Export matches to CSV.vi"("Score"=w225, "PosY"=w226, "PosX"=w227, "filenames for processing"=w224, "Data Export Filepath"=w223) -> ()  [unwired: 7 in]
        n97 = call <vilib>:"Add State(s) to Queue__jki_lib_state_machine.vi"("State(s) in (\"\")"=w231) -> ("States Out"=w230:string)  [unwired: 14 in]
      }
      frame "---------- UI ----------" {
        # "Do not put any code in this frame.\n(It is a separator no-op. You can make a copy of this frame to create a new UI frame)"
        n98 = call <vilib>:"Add State(s) to Queue__jki_lib_state_machine.vi"("State(s) in (\"\")"=w235) -> ("States Out"=w234:string)  [unwired: 14 in]
      }
      frame "UI: Update Match Result" {
        n99 = Unbundle By Name(w243) -> ("PosX"=w242:sgl[], "PosY"=w237:sgl[], "Score"=w238:sgl[])
        n100 = property on="Source Images" class="Arr (strict)"() -> ("Array Element.Value"=w245:variant, "Index Values"=w244:u32[])  [unwired: 2 in, 2 out]
        n101 = Index Array(array=w244) -> (element=w236:u32)  [unwired: 1 in]
        n102 = local write "Filename"(w245) -> ()
        n103 = Index Array(array=w242, index=w236) -> (element=→"Position.x":sgl)
        n104 = Index Array(array=w237, index=w236) -> (element=→"Position.y":sgl)
        n105 = Index Array(array=w238, index=w236) -> (element=→"Score":sgl)
        n106 = call <vilib>:"Add State(s) to Queue__jki_lib_state_machine.vi"("State(s) in (\"\")"=w248) -> ("States Out"=w247:string)  [unwired: 14 in]
      }
      frame "UI: Initialize" {
        # "Initialize the User Interface, here.\n(this is called automatically, by the Macro: Init)"
        n107 = call <vilib>:"Add State(s) to Queue__jki_lib_state_machine.vi"("State(s) in (\"\")"=w252) -> ("States Out"=w251:string)  [unwired: 14 in]
      }
      frame "UI: Cursor Set" {
        # "Argument"
        # "Set and Unset Cursor Busy.\n(Usage: \"UI: Cursor Set >> Busy|Idle\")"
        n108 = case shown="\"Busy\"" w253 {
          tunnel: w255 -> [w260 w262]
          tunnel: [w259 w261] -> w254
          frame "Idle", Default {
            n109 = call <vilib>:"Unset Busy.vi"("error in (no error)"=w260) -> ("error out"=w259:errorcluster)  [unwired: 10 in]
          }
          frame "Busy" {
            n110 = call <vilib>:"Set Busy.vi"("error in (no error)"=w262) -> ("error out"=w261:errorcluster)  [unwired: 9 in, 1 out]
          }
        }
        n111 = call <vilib>:"Add State(s) to Queue__jki_lib_state_machine.vi"("State(s) in (\"\")"=w258) -> ("States Out"=w257:string)  [unwired: 14 in]
      }
      frame "UI: Front Panel State" {
        # "Argument"
        # "Set Front Panel Open or Closed\n(Usage: \"UI: Front Panel State >> Open|Close\")"
        n112 = Unbundle By Name(w265) -> ("Core.Current VI Reference"=w264:refnum<vi>)
        n113 = case shown="\"Open\", Default" w263 {
          tunnel: w267 -> [w273 w286]
          tunnel: [w275 w287] -> w266
          tunnel: w264 -> [w274 w284]
          frame "Open", Default {
            n114 = property class="VI"(reference=w274, error in=w273) -> (reference out=w271:refnum<vi>, error out=w272:errorcluster, "Front Panel.Open"=w270:bool)
            n115 = case shown="False" w270 {
              tunnel: [w278 w281] -> w275
              tunnel: w272 -> [w277 w281]
              tunnel: w271 -> [w276 _]
              frame False {
                n116 = invoke class="VI" method="FP.Open"(reference=w276, error in=w277, "Activate"=TRUE, "State"=T3."Standard") -> (error out=w278:errorcluster)  [unwired: 1 in, 4 out]
              }
              frame True {
              }
            }
          }
          frame "Close" {
            n117 = property class="VI"(reference=w284, error in=w286) -> (reference out=w283:refnum<vi>, error out=w285:errorcluster, "Front Panel.Open"=w282:bool)
            n118 = case shown="True" w282 {
              tunnel: [w288 w291] -> w287
              tunnel: w285 -> [w288 w290]
              tunnel: w283 -> [_ w289]
              frame False {
              }
              frame True {
                n119 = invoke class="VI" method="FP.Close"(reference=w289, error in=w290) -> (error out=w291:errorcluster)  [unwired: 1 in, 2 out]
              }
            }
          }
        }
        n120 = call <vilib>:"Add State(s) to Queue__jki_lib_state_machine.vi"("State(s) in (\"\")"=w269) -> ("States Out"=w268:string)  [unwired: 14 in]
      }
      frame "---------- Macro ----------" {
        # "Do not put any code in this frame.\n(It is a separator no-op. You can make a copy of this frame to create a new Macro frame)"
        n121 = call <vilib>:"Add State(s) to Queue__jki_lib_state_machine.vi"("State(s) in (\"\")"=w295) -> ("States Out"=w294:string)  [unwired: 14 in]
      }
      frame "Macro: Initialize" {
        w296 = "Data: Initialize\nInitialize Core Data\nUI: Initialize\nData: Clear Match Results\nUI: Front Panel State >> Open"  # Data: Initialize Initialize Core Data UI: Initialize Data: Clear Match Results UI: Front Panel State >> Open
        # "Initialization Macro\n(This is called once, when the VI starts)"
        n122 = call <vilib>:"Add State(s) to Queue__jki_lib_state_machine.vi"("State(s) in Front (\"\")"=w296, "State(s) in (\"\")"=w300) -> ("States Out"=w299:string)  [unwired: 13 in]
      }
      frame "Macro: Exit" {
        # "Exit Macro\n(This is called once, when the VI exits)"
        n123 = Unbundle By Name(w307) -> ("Core.Close Panel on Exit?"=w306:bool)
        n124 = Select(t="UI: Front Panel State >> Close", s=w306, f="") -> (s? t:f=w303:string)
        n125 = call <vilib>:"Add State(s) to Queue__jki_lib_state_machine.vi"("State(s) in (\"\")"=w303, "State(s) at Back (\"\")"="Data: Cleanup\nExit") -> ("States Out"=w301:string)  [unwired: 13 in]
        n126 = call <vilib>:"Add State(s) to Queue__jki_lib_state_machine.vi"("State(s) in Front (\"\")"=w301, "State(s) in (\"\")"=w310) -> ("States Out"=w309:string)  [unwired: 13 in]
      }
      frame "---------- Image ----------" {
        # "Template Separator\n(You can make a copy of, or modify, this frame)"
        n127 = call <vilib>:"Add State(s) to Queue__jki_lib_state_machine.vi"("State(s) in (\"\")"=w314) -> ("States Out"=w313:string)  [unwired: 14 in]
      }
      frame "Image: PatternFind all Images" {
        w319 = T6 0 items=["Grayscale (U8)", "Grayscale (I16)", "Grayscale (SGL)", "Complex (CSG)", "RGB (U32)", "HSL (U32)", "RGB (U64)", "Grayscale (U16)"] ("Image Type")
        n128 = Unbundle By Name(w331) -> ("FiducialImages"=w326:T1[], "PatternTemplate"=w332:T1, "ImageResults"=w330:T1)
        n129 = Bundle By Name(cluster=T4 {"Match Mode"=1, "Number of Matches Requested"=1, "Minimum Match Score"=800.0, "SubPixel Accuracy"=TRUE, "Rotation Angle Ranges"=[], "Show Search Area"=FALSE, "Show Result"=TRUE} ("Settings"), "Minimum Match Score"="Minimum Match Score", "Rotation Angle Ranges"="Rotation Angle \nSearch Ranges") -> (w320:T4)
        n130 = call "IMAQ Create"("Image Name"="asdfasdfsdf", "Image Type"=w319) -> ("New Image"=w317:T1)  [unwired: 3 in, 1 out]
        n131 = for {
          tunnel: w326 -> [w346] mode=indexing
          tunnel: w332 -> [w359]
          tunnel: w330 -> [w360]
          shift-right: [w340] -> w325
          shift-left: w333 -> [w347]
          shift-right: [w355] -> w329
          shift-left: w331 -> [w356]
          tunnel: w320 -> [w344]
          tunnel: w317 -> [_]
          tunnel: "Size" -> [w339]
          tunnel: "Overlay Color" -> [w338]
          i -> [w353]
          # "find pattern"
          n132 = call "IMAQ Find Pattern 3"("Settings"=w344, "Template"=w359, "error in (no error)"=w347, "Image"=w346) -> ("error out"=w352:errorcluster, "Image Out"=w337:T1, "Matches"=w358:T8)  [unwired: 2 in, 3 out]
          n133 = Index Array(array=w358) -> (element=w357:T9)  [unwired: 1 in]
          n134 = Unbundle By Name(w357) -> ("Score"=w345:sgl, "Position.x"=w349:sgl, "Position.y"=w348:sgl, "Bounding Box"=w343:cluster{"x":sgl, "y":sgl}[])
          n135 = Greater Than 0?(x=w353) -> (x > 0?=w354:bool)
          n136 = case "1st image as background" shown="False" w354 {
            tunnel: w352 -> [w367 w368]
            tunnel: [w361 w368] -> w342
            tunnel: w360 -> [w366 w369]
            tunnel: [w363 w369] -> w351
            tunnel: w337 -> [w365 _]
            frame False {
              n137 = call "IMAQ Copy"("error in (no error)"=w367, "Image Dst"=w366, "Image Src"=w365) -> ("error out"=w362:errorcluster, "Image Dst Out"=w364:T1)  [unwired: 3 in]
              n138 = call "IMAQ Clear Overlay"("error in (no error)"=w362, "Image"=w364) -> ("error out"=w361:errorcluster, "Image Out"=w363:T1)  [unwired: 8 in]
            }
            frame True {
            }
          }
          n139 = in-place "Record results" {
            in-place-border: w349 -> [w377]
            in-place-border: w348 -> [w375]
            in-place-border: w345 -> [w372]
            n140 = in-place-cluster #2(w356) -> ("PosX"=w378:sgl[], "PosY"=w376:sgl[], "Score"=w370:sgl[])
            n141 = Build Array (concatenate)(w378, w377) -> (w373:sgl[])
            n142 = Build Array (concatenate)(w376, w375) -> (w374:sgl[])
            n143 = Build Array (concatenate)(w370, w372) -> (w371:sgl[])
            n144 = in-place-cluster #2("PosX"=w373, "PosY"=w374, "Score"=w371) -> (w355:T5)
          }
          n145 = call "Draw Dot.vi"("Color"=w338, "CenterX"=w349, "error in (no error)"=w342, "Size"=w339, "CenterY"=w348, "Refnum in"=w351) -> ("error out"=w341:errorcluster, "Refnum out"=w350:T1)  [unwired: 4 in]
          n146 = local write "All Results"(w350) -> ()
          n147 = call "Crop to Bounding Box.vi"("error in (no error)"=w341, "Bounding Box"=w343, "Refnum in"=w337) -> ("error out"=w340:errorcluster)  [unwired: 8 in]
        }
        n148 = Unbundle By Name(w329) -> ("PosX"=→"PosX":sgl[], "PosY"=→"PosY":sgl[], "Score"=→"Score all":sgl[])
        n149 = flat-sequence {
          tunnel: w326 -> [w336]
          tunnel: w325 -> [_]
          frame #0 {
            n150 = local write "Source Images"(w336) -> ()
          }
        }
        n151 = call <vilib>:"Add State(s) to Queue__jki_lib_state_machine.vi"("State(s) in (\"\")"=w335) -> ("States Out"=w334:string)  [unwired: 14 in]
      }
    }
  }
